vi "BitUnPacking.vi"(7 "Bits":u8=12, 10 "Pixels":i32=3, 11 "ByteArray":u8[](array[numeric])=[18, 53, 103, 154, 176] format="%02x") -> (3 "Array":u16[](array[numeric]) format="%04x")   [LabVIEW 2011]
panel:
  out "Bytes":u32
  out "Pixel":u32
  # "größer out:15bytes; 15bit 8zu15, 8byte ginge in U64\ngrößter in:8Pixel; 1,3,5,7,9,11,13.15 bit 8zu x"
  # "no offset alyways msb!"
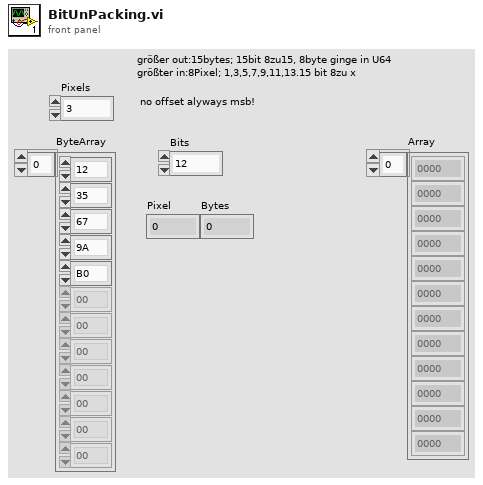
[diagram p1: front panel]
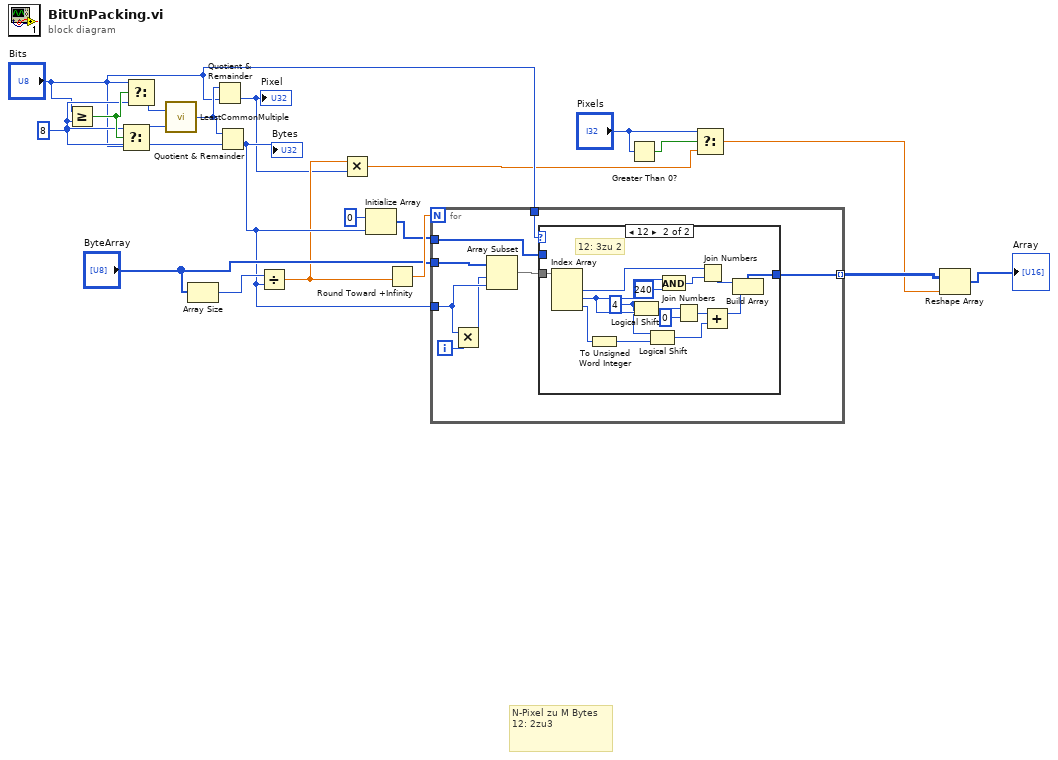
[diagram p0: block diagram]
diagram:
  w16 = u32 8 ("Numeric (larger)")
  # "N-Pixel zu M Bytes\n12: 2zu3"
  n1 = Greater Or Equal?(x="Bits", y=w16) -> (x >= y?=w18:bool)
  n2 = Select(t=w16, s=w18, f="Bits") -> (s? t:f=w19:u32)
  n3 = Select(t="Bits", s=w18, f=w16) -> (s? t:f=w20:u32)
  n4 = call "LeastCommonMultiple.vi"("Numeric (larger)"=w19, "Numeric"=w20) -> ("LCM"=w17:u32)
  n5 = Array Size(array="ByteArray") -> (size(s)=w9:i32)
  n6 = Quotient & Remainder(x=w17, y="Bits") -> (floor(x/y)=w2:u32)  [unwired: 1 out]
  "Pixel" <- w2
  n7 = Quotient & Remainder(x=w17, y=w16) -> (floor(x/y)=w8:u32)  [unwired: 1 out]
  "Bytes" <- w8
  n8 = Divide(x=w9, y=w8) -> (x/y=w3:dbl)
  n9 = Multiply(x=w3, y=w2) -> (x*y=w1:dbl)
  n10 = Initialize Array(u8 0 ("element"), w8) -> (w13:u8[])
  n11 = Round Toward +Infinity(x=w3) -> (ceil(x): smallest int >= x=w15:dbl)
  n12 = for {
    N: w15 -> [_]
    tunnel: "ByteArray" -> [w28]
    tunnel: w8 -> [w26]
    tunnel: w13 -> [w21]
    tunnel: "Bits" -> [w23]
    tunnel: [w22] -> w11 mode=indexing
    i -> [w27]
    n13 = Multiply(x=w26, y=w27) -> (x*y=w25:u32)
    n14 = Array Subset(array=w28, index=w25, length=w26) -> (w24:u8[])
    n15 = case shown="12" w23 {
      tunnel: w24 -> [_ w44]
      tunnel: [w29 w43] -> w22
      tunnel: w21 -> [w29 _]
      frame 0, Default {
      }
      frame 12 {
        w33 = i8 4 ("y")
        # "12: 3zu 2"
        n16 = Index Array(array=w44) -> (element #1=w40:u8, element #2=w37:u8, element #3=w35:u8)  [unwired: 3 in]
        n17 = To Unsigned Word Integer(number=w35) -> (unsigned 16bit integer=w34:u16)
        n18 = Logical Shift(y=w33, x=w37) -> (x << y=w36:u8)
        n19 = Logical Shift(y=w33, x=w34) -> (x << y=w30:u16)
        n20 = And(x=w37, y=u8 240) -> (x .and. y?=w38:u8)
        n21 = Join Numbers(hi=w36, lo=u8 0) -> ((hi.lo)=w41:u16)
        n22 = Join Numbers(hi=w40, lo=w38) -> ((hi.lo)=w42:u16)
        n23 = Add(x=w41, y=w30) -> (x+y=w31:u16)
        n24 = Build Array(w42, w31) -> (w43:u16[])
      }
    }
  }
  n25 = Greater Than 0?(x="Pixels") -> (x > 0?=w4:bool)
  n26 = Select(t="Pixels", s=w4, f=w1) -> (s? t:f=w5:dbl)
  n27 = Reshape Array(w11, w5) -> (→"Array":u16[])
